vi "Stop Core.vi"(10 "final error code":i32, 11 "Devices to Load in":refnum<class "Devices to Load.lvclass">) -> (3 "Devices to Load out":refnum<class "Devices to Load.lvclass">)   [LabVIEW 2018, in "Devices to Load Config Actor.lvlib" / "Devices to Load.lvclass"]
doc: "(<B>Filename</B>: Actor Framework.lvlib:Actor.lvclass:Stop Core.vi)\n\nDefines what the actor does before it stops. Use the <B>final error code</B> input to determine whether the actor shut down in response to an error.\n\nBy default, this method does nothing. A descendant class may override it to define behavior, such as shutting down any processes the actor initiated in its override of the Actor Core method."
uses:
  Devices to Load.lvclass
  Devices to Load.lvclass/Devices to Load.ctl
  <vilib>/ActorFramework/Actor/Actor.lvclass
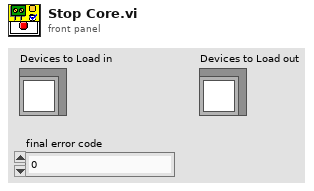
[diagram p1: front panel]
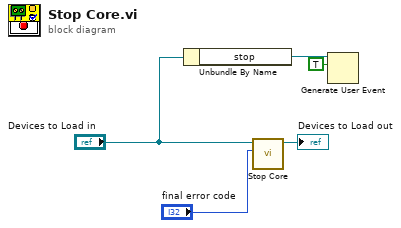
[diagram p0: block diagram]
diagram:
  n1 = Unbundle By Name("Devices to Load in") -> ("stop"=w2:refnum<user-event>)
  n2 = call-parent "Stop Core.vi"("final error code"="final error code", "Actor in"="Devices to Load in") -> ("Actor out"=→"Devices to Load out":refnum<class "Devices to Load.lvclass">)  [unwired: 9 in]
  n3 = Generate User Event(user event=w2, event data cluster=TRUE ("event data")) -> ()  [unwired: 2 in, 2 out]
